vi "Add_to_Cost_Func_Addition_from_Subtrk-1.vi"(2 "[IN] Cost function":i8[](array[numeric]), 3 "[IN] Subtracks in Row":T1(array[cluster])) -> (0 "[OUT] Cost function":i8[](array[numeric]))   [LabVIEW 2017]
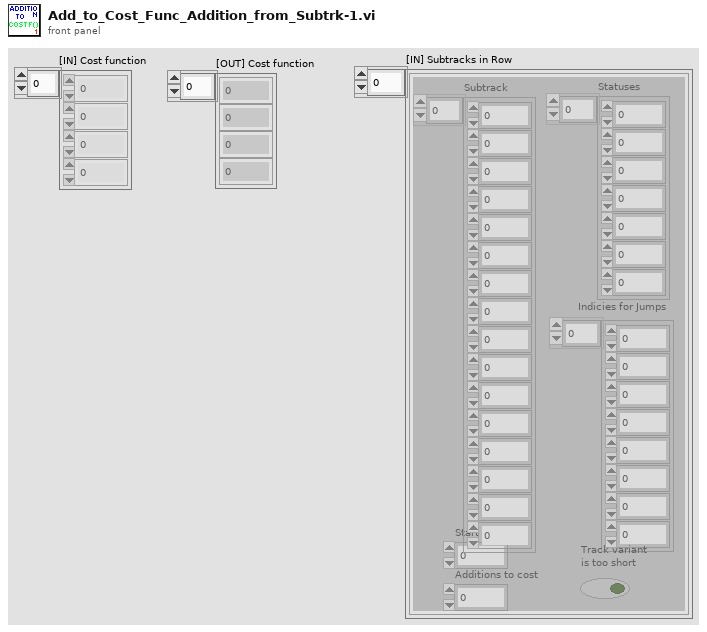
[diagram p1: front panel]
types:
  T1 = cluster{"Subtrack":dbl[], "Statuses":i16[], "Start pos":i32, "Additions to cost":i8, "Track variant \nis too short":bool, "Indicies for Jumps":i32[]}[]
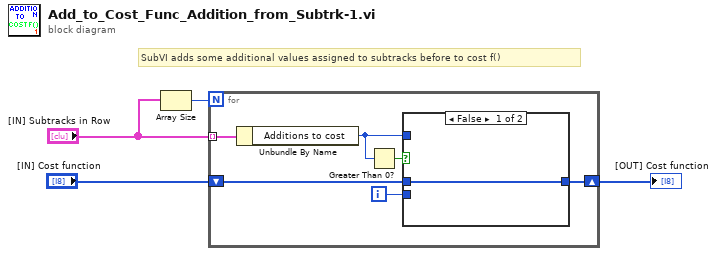
[diagram p0: block diagram]
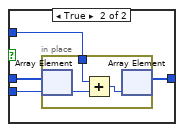
[diagram p2: hidden frame]
diagram:
  # "SubVI adds some additional values assigned to subtracks before to cost f()"
  n1 = Array Size(array="[IN] Subtracks in Row") -> (size(s)=w4:i32)
  n2 = for {
    N: w4 -> [_]
    tunnel: "[IN] Subtracks in Row" -> [w10] mode=indexing
    shift-right: [w7] -> w1
    shift-left: "[IN] Cost function" -> [w9]
    i -> [w8]
    n3 = Unbundle By Name(w10) -> ("Additions to cost"=w5:i8)
    n4 = Greater Than 0?(x=w5) -> (x > 0?=w6:bool)
    n5 = case shown="False" w6 {
      tunnel: w9 -> [w11 w15]
      tunnel: w8 -> [_ w14]
      tunnel: w5 -> [_ w13]
      tunnel: [w11 w12] -> w7
      frame False {
      }
      frame True {
        n6 = in-place {
          in-place-border: w13 -> [w17]
          n7 = in-place-array #1(w15, w14) -> (w18:i8)
          n8 = Add(x=w17, y=w18) -> (x+y=w16:i8)
          n9 = in-place-array #1(w16) -> (w12:i8[])  [unwired: 1 out]
        }
      }
    }
  }
  "[OUT] Cost function" <- w1
